vi "Create.vi"(6 "Priority (normal)":T1=enum."normal priority", 8 "error in (no error)":errorcluster, 9 "Reply Channel":refnum<notifier>, 10 "Data":variant, 11 "Name":string) -> (0 "error out":errorcluster, 3 "Message out":refnum<class "Message.lvclass">)   [LabVIEW 2015, in "Message.lvclass"]
uses:
  Message.lvclass
  <vilib>/event_ctls.llb/usereventprio.ctl
  Message.lvclass/Message.ctl
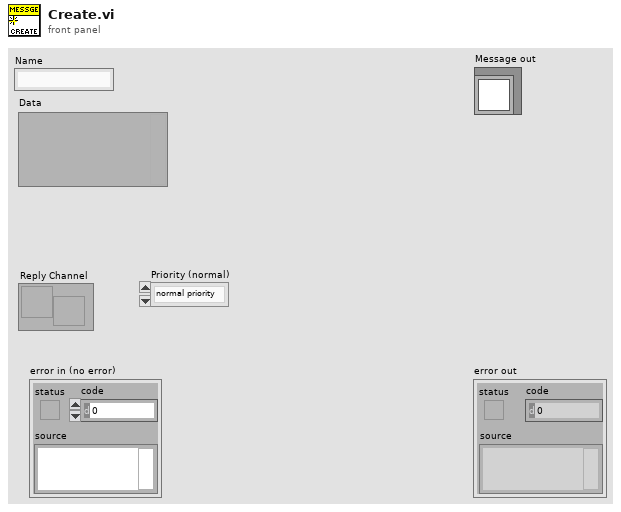
[diagram p1: front panel]
types:
  T1 = typedef "usereventprio.ctl" = enum32{"high priority", "normal priority"}
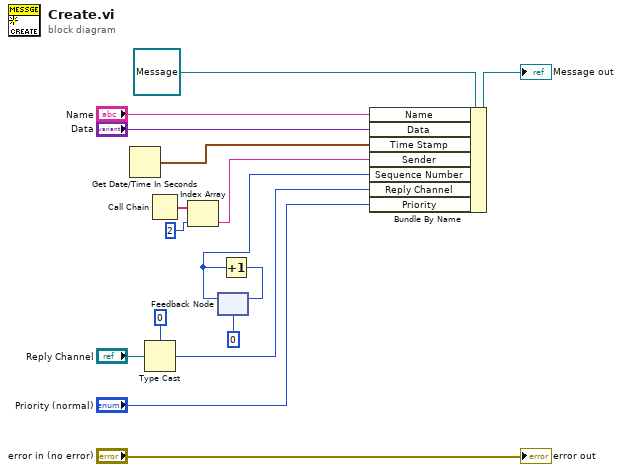
[diagram p0: block diagram]
diagram:
  n1 = Get Date/Time In Seconds() -> (seconds since 1Jan1904=w10:timestamp)
  n2 = Type Cast(type=u32 0 ("Reply Channel"), x="Reply Channel") -> (*(type *) &x=w5:u32)
  n3 = Call Chain() -> (call chain=w3:string[])
  n4 = Index Array(array=w3, index=2 ("Index")) -> (element=w2:string)
  n5 = feedback #1(u64 0) -> (w8:u64)
  n6 = Increment(x=w8) -> (x+1=w9:u64)
  n7 = feedback-in #1(w9) -> ()
  n8 = Bundle By Name(cluster=refnum<class "Message.lvclass"> refnum ("Message in"), "Name"="Name", "Data"="Data", "Time Stamp"=w10, "Sender"=w2, "Sequence Number"=w8, "Reply Channel"=w5, "Priority"="Priority (normal)") -> (→"Message out":refnum<class "Message.lvclass">)
  "error out" <- "error in (no error)"
